vi "Abort.vi"(8 "error in (no error)":errorcluster, 11 "Test Runner In":refnum<class "Test Runner.lvclass">) -> (0 "error out":errorcluster, 3 "Test Runner Out":refnum<class "Test Runner.lvclass">)   [LabVIEW 2020, in "Test Runner.lvclass"]
uses:
  Test Runner.lvclass
  Test Runner.lvclass/Test Runner.ctl
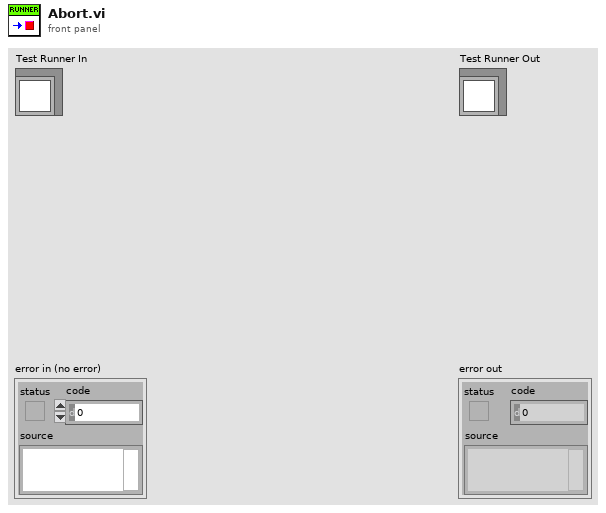
[diagram p1: front panel]
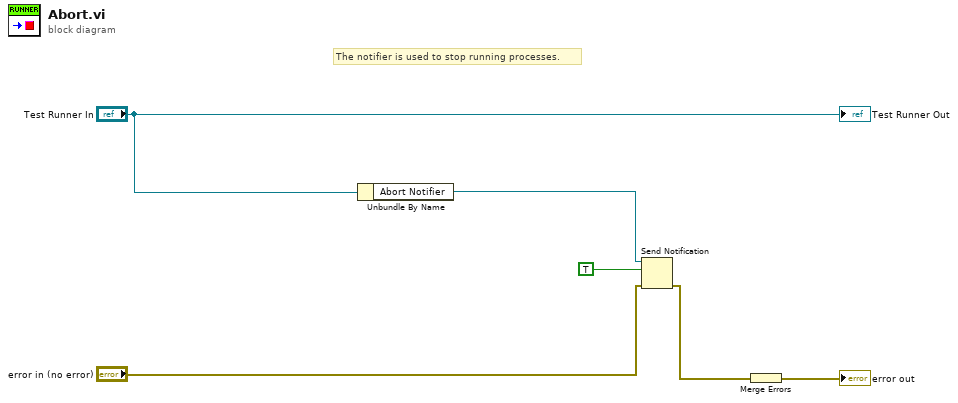
[diagram p0: block diagram]
diagram:
  # "The notifier is used to stop running processes."
  n1 = Unbundle By Name("Test Runner In") -> ("Abort Notifier"=w6:refnum<notifier>)
  n2 = Send Notification(notification=TRUE, notifier=w6, error in (no error)="error in (no error)") -> (error out=w2:errorcluster)  [unwired: 1 out]
  n3 = Merge Errors(w2) -> (→"error out":errorcluster)
  "Test Runner Out" <- "Test Runner In"
